vi "Destroy Thread.vi"(8 "error in (no error)":errorcluster, 11 "Thread in":refnum<class "Thread.lvclass">) -> (0 "error out":errorcluster)   [LabVIEW 2013, in "Architecture.lvlib" / "Thread.lvclass"]
uses:
  Thread.lvclass
  Queue.lvclass
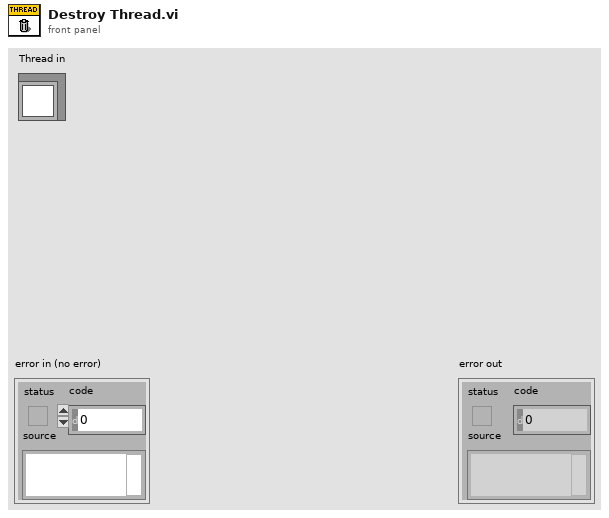
[diagram p1: front panel]
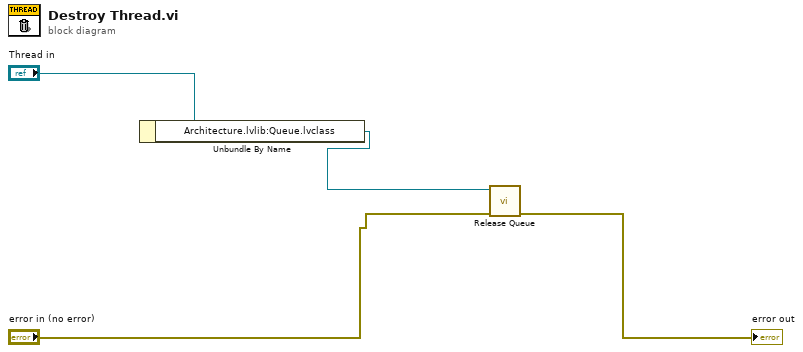
[diagram p0: block diagram]
diagram:
  n1 = Unbundle By Name("Thread in") -> ("Architecture.lvlib:Queue.lvclass"=w3:refnum<class "Queue.lvclass">)
  n2 = call "Release Queue.vi"("error in (no error)"="error in (no error)", "Queue in"=w3) -> ("error out"=→"error out":errorcluster)  [unwired: 8 in, 1 out]
